vi "ASE.vi"(4 "Position":cluster{"X":sgl, "Y":sgl, "Z":sgl}, 8 "error in (no error)":errorcluster, 9 "Model File":path, 10 "Name":string) -> (0 "error out":errorcluster, 3 "Object out":refnum<class "3D Object.lvclass">)   [LabVIEW 2015, in "3D Object.lvclass"]
uses:
  3D Object.lvclass
  <vilib>/picture/3D Picture Control/NI_3D Picture Control.lvlib
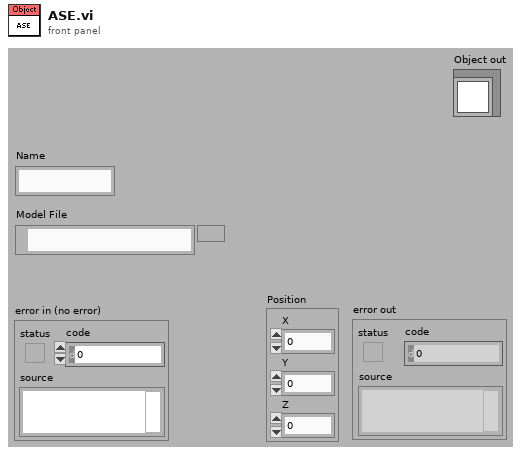
[diagram p1: front panel]
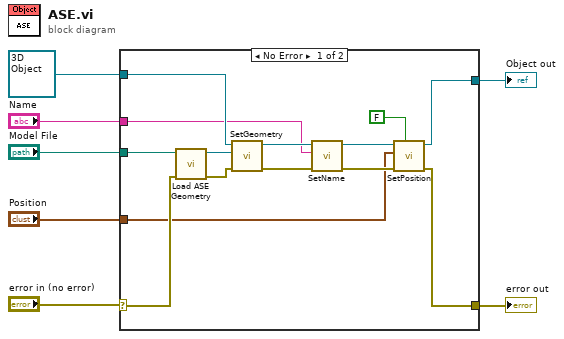
[diagram p0: block diagram]
diagram:
  n1 = case shown="No Error" "error in (no error)" {
    selector: "error in (no error)" -> [w10 w23]
    tunnel: "Model File" -> [w21 _]
    tunnel: refnum<class "3D Object.lvclass"> refnum ("Object in") -> [w16 w22]
    tunnel: [w19 w22] -> w4
    tunnel: [w18 w23] -> w3
    tunnel: "Position" -> [w9 _]
    tunnel: "Name" -> [w15 _]
    frame No Error {
      n2 = call <vilib>:"Load ASE Geometry.vi"("error in (no error)"=w10, "Model File"=w21) -> ("error out"=w13:errorcluster, "New Mesh Refnum"=w20:refnum<vi>)  [unwired: 8 out]
      n3 = call "SetGeometry.vi"("error in (no error)"=w13, "Geometry"=w20, "Object in"=w16) -> ("error out"=w14:errorcluster, "Object out"=w17:refnum<class "3D Object.lvclass">)  [unwired: 7 out]
      n4 = call "SetName.vi"("error in (no error)"=w14, "Name"=w15, "3D Object in"=w17) -> ("error out"=w12:errorcluster, "3D Object out"=w11:refnum<class "3D Object.lvclass">)  [unwired: 7 out]
      n5 = call "SetPosition.vi"("Relative?"=FALSE, "error in (no error)"=w12, "Position"=w9, "3D Object in"=w11) -> ("error out"=w18:errorcluster, "3D Object out"=w19:refnum<class "3D Object.lvclass">)  [unwired: 6 in]
    }
    frame Error {
    }
  }
  "error out" <- w3
  "Object out" <- w4
